vi "TCP Listen Internal List.vi"(5 "net address":u32, 7 "service name":string, 8 "Index #":i32, 9 "Element In":T1, 10 "Port":u16, 11 "Operation":T2) -> (0 "Element # \n(-1 if not found)":i32, 2 "Conflict":bool, 3 "Item Requested":T1)   [LabVIEW 2017]
uses:
  <vilib>/Utility/tcp.llb/TCP Listen List Operations.ctl
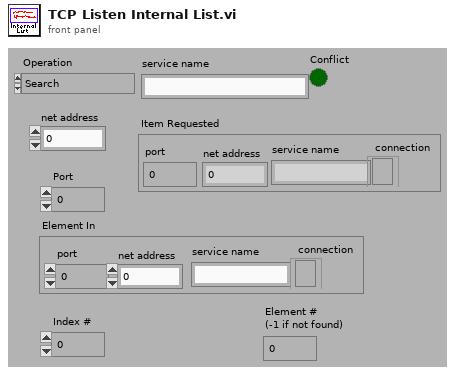
[diagram p1: front panel]
types:
  T1 = cluster{"port":u16, "service name":string, "connection":refnum<k5>, "net address":u32}
  T2 = typedef "TCP Listen List Operations.ctl" = enum16{"Search", "Retrieve Element", "Add Element", "Delete Element"}
  T3 = cluster{"port":u16, "service name":string, "connection":refnum<k5>, "net address":u32}[]
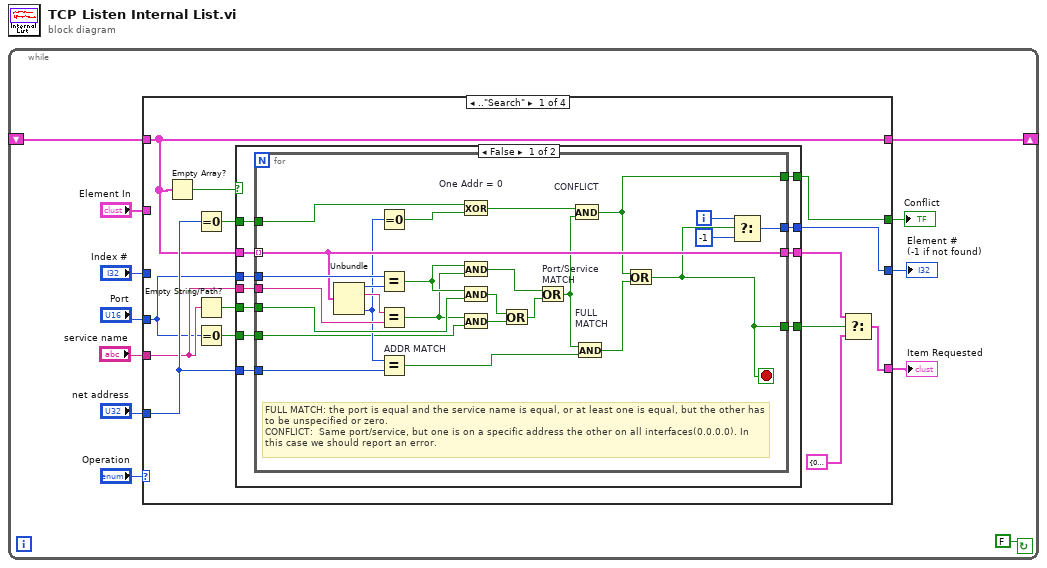
[diagram p0: block diagram]
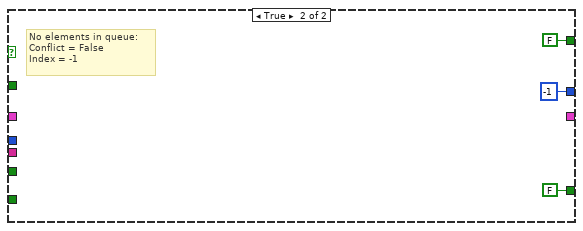
[diagram p2: hidden frame]
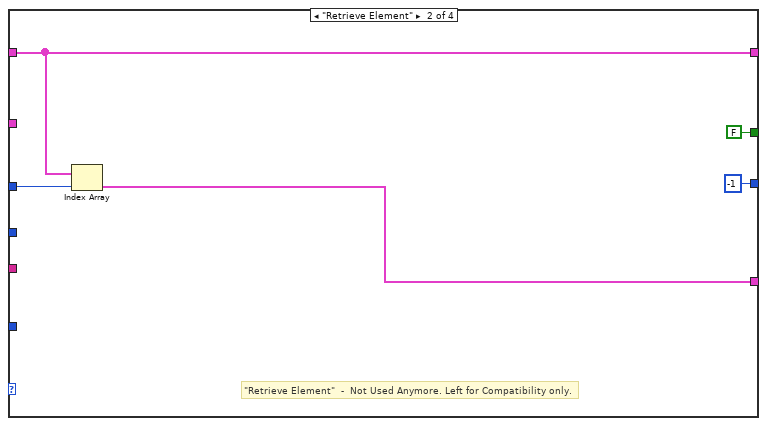
[diagram p3: hidden frame]
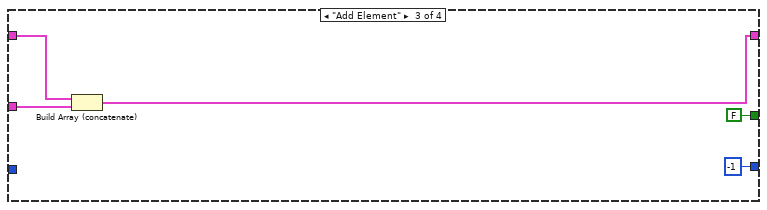
[diagram p4: hidden frame]
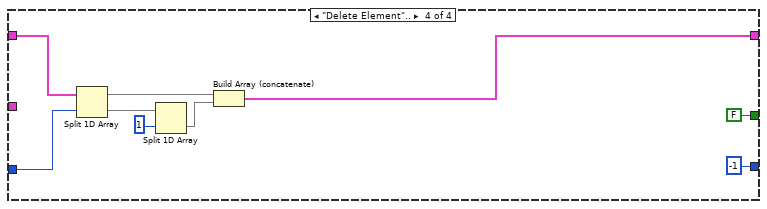
[diagram p5: hidden frame]
diagram:
  n1 = while {
    shift-left: _ -> [w10]
    shift-right: [w8] -> _
    stop <- FALSE continue-if-true
    n2 = case shown="..\"Search\"" "Operation" {
      tunnel: "Element In" -> [_ _ w75 _]
      tunnel: "Index #" -> [_ w71 _ w85]
      tunnel: w10 -> [w15 w70 w76 w84]
      tunnel: "Port" -> [w17 _ _ _]
      tunnel: [w15 w70 w74 w79] -> w8
      tunnel: [w25 -1 ("f") -1 ("f") -1] -> w6
      tunnel: [w22 w69 _ _] -> w2
      tunnel: "service name" -> [w19 _ _ _]
      tunnel: "net address" -> [w26 _ _ _]
      tunnel: [w20 FALSE FALSE FALSE] -> w1
      frame .."Search" {
        n3 = Empty Array?(array=w15) -> (empty?=w14:bool)
        n4 = Equal To 0?(x=w26) -> (x = 0?=w24:bool)
        n5 = Empty String/Path?(string/path=w19) -> (empty?=w18:bool)
        n6 = Equal To 0?(x=w17) -> (x = 0?=w16:bool)
        n7 = case shown="False" w14 {
          tunnel: w26 -> [w37 _]
          tunnel: [w36 -1 ("f")] -> w25
          tunnel: w24 -> [w35 _]
          tunnel: [w34 _] -> w23
          tunnel: [w33 FALSE] -> w21
          tunnel: [w32 FALSE] -> w20
          tunnel: w15 -> [w31 _]
          tunnel: w19 -> [w30 _]
          tunnel: w18 -> [w29 _]
          tunnel: w17 -> [w28 _]
          tunnel: w16 -> [w27 _]
          frame False {
            n8 = for {
              tunnel: w31 -> [w53] mode=indexing
              tunnel: w28 -> [w63]
              tunnel: w30 -> [w60]
              tunnel: w27 -> [w44]
              tunnel: w29 -> [w59]
              tunnel: w37 -> [w46]
              tunnel: [w53] -> w34
              tunnel: w35 -> [w51]
              tunnel: [w38] -> w33
              tunnel: [w48] -> w36
              tunnel: [w39] -> w32
              i -> [w40]
              stop <- w38 stop-if-true
              # "FULL MATCH: the port is equal and the service name is equal, or at least one is equal, but the other has to be unspecified or zero. \nCONFLICT:  Same port/service, but one is on a specific address the other on all interfaces(0.0.0.0). In this case we should report an error."
              n9 = Unbundle(w53) -> ("port"=w62:u16, "service name"=w61:string, "net address"=w45:u32)  [unwired: 1 out]
              n10 = Equal To 0?(x=w45) -> (x = 0?=w52:bool)
              n11 = Equal?(x=w63, y=w62) -> (x = y?=w58:bool)
              n12 = Equal?(x=w61, y=w60) -> (x = y?=w43:bool)
              n13 = Equal? "ADDR MATCH"(x=w45, y=w46) -> (x = y?=w49:bool)
              n14 = Exclusive Or "One Addr = 0"(1:w52, 2:w51) -> (0:w50:bool)
              n15 = And(x=w58, y=w43) -> (x .and. y?=w54:bool)
              n16 = And(x=w58, y=w59) -> (x .and. y?=w56:bool)
              n17 = And(x=w43, y=w44) -> (x .and. y?=w57:bool)
              n18 = Or(x=w56, y=w57) -> (x .or. y?=w55:bool)
              n19 = Or "Port/Service\nMATCH"(x=w54, y=w55) -> (x .or. y?=w47:bool)
              n20 = And "CONFLICT"(x=w50, y=w47) -> (x .and. y?=w39:bool)
              n21 = And "FULL \nMATCH"(x=w47, y=w49) -> (x .and. y?=w42:bool)
              n22 = Or(x=w39, y=w42) -> (x .or. y?=w38:bool)
              n23 = Select(t=w40, s=w38, f=-1) -> (s? t:f=w48:i32)
            }
          }
          frame True {
            # "No elements in queue:  \nConflict = False\nIndex = -1"
          }
        }
        n24 = Select(t=w23, s=w21, f=T1 {"port"=0, "service name"="", "connection"=refnum, "net address"=0}) -> (s? t:f=w22:T1)
      }
      frame "Retrieve Element" {
        # "\"Retrieve Element\"  -  Not Used Anymore. Left for Compatibility only."
        n25 = Index Array(array=w70, index=w71) -> (element=w69:T1)
      }
      frame "Add Element" {
        n26 = Build Array (concatenate)(w76, w75) -> (w74:T3)
      }
      frame "Delete Element".. {
        n27 = Split 1D Array(array=w84, index=w85) -> (first subarray=w80:T3, second subarray=w82:T3)
        n28 = Split 1D Array(array=w82, index=1) -> (second subarray=w81:T3)  [unwired: 1 out]
        n29 = Build Array (concatenate)(w80, w81) -> (w79:T3)
      }
    }
    "Element # \n(-1 if not found)" <- w6
    "Item Requested" <- w2
    "Conflict" <- w1
  }
